vi "Run Tests.vi"(7 "Run Tests In Parallel? (T)":bool=TRUE, 8 "error in (no error)":errorcluster, 10 "Report Output path":path, 11 "Project, Library, or Test Class Path":path) -> (0 "error out":errorcluster, 1 "All Passed?":bool, 2 "Output":string)   [LabVIEW 2020, in "Execution API.lvclass"]
doc: "Run all tests from the selected path programmatically. The path may point to a .lvclass, .lvlib, or .lvproj file. Results are generated at the provided Report Output Path. If the file extenssion is .txt, a plain text file is generated, and if it is .xml, an JUnit compatible .xml report is generated."
uses:
  Execution API.lvclass
  Core/Result/Status.ctl
  Core/Result/Type.ctl
  Core/Result/Result.lvlib
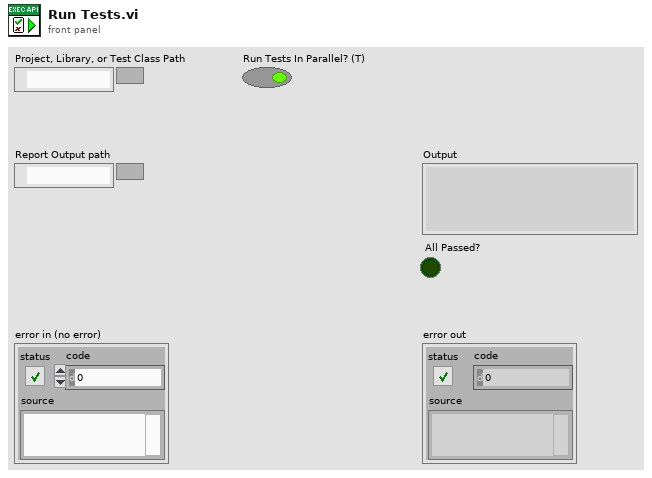
[diagram p1: front panel]
types:
  T1 = typedef "Result.lvlib/Status.ctl" = enum16{"", "Passed", "Failed", "Error", "Skipped", "Setup Error", "Broken", "Teardown Error"}
  T2 = typedef "Result.lvlib/Type.ctl" = enum16{"Test Case", "Test Suite", "Test Run", "Pass", "Fail", "Skip", "Pass if", "Fail if", "Pass if Error", "Fail if Error", "Pass if Equal", "Fail if Equal"}
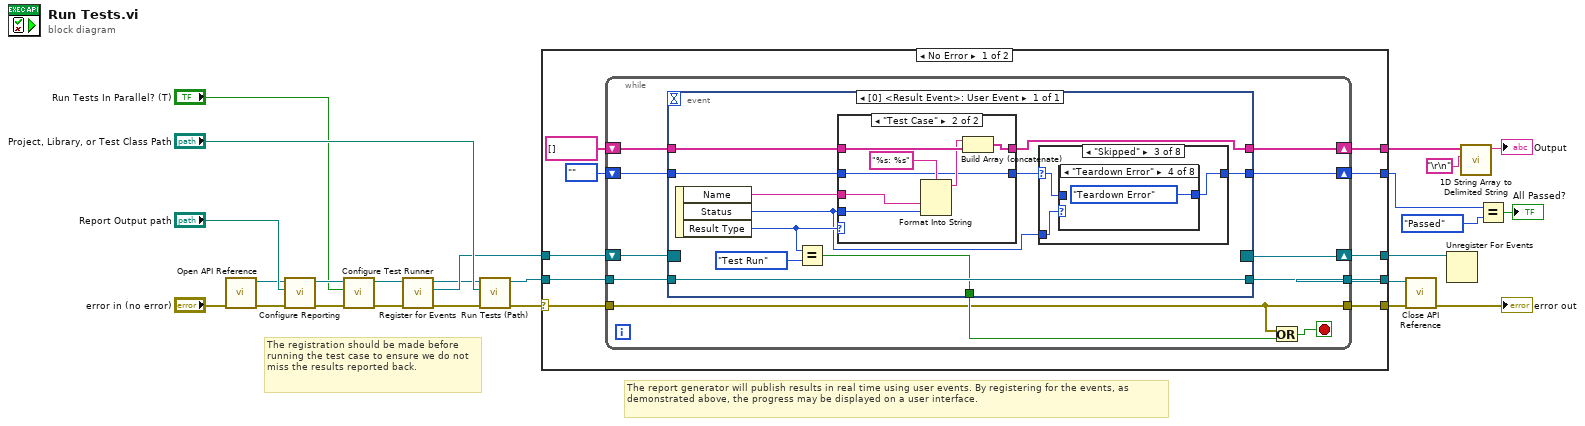
[diagram p0: block diagram]
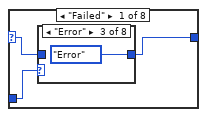
[diagram p3: hidden frame]
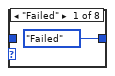
[diagram p4: hidden frame]
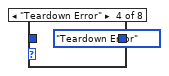
[diagram p6: hidden frame]
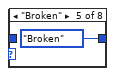
[diagram p7: hidden frame]
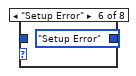
[diagram p8: hidden frame]
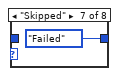
[diagram p9: hidden frame]
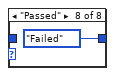
[diagram p10: hidden frame]
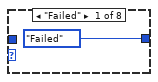
[diagram p12: hidden frame]
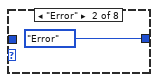
[diagram p13: hidden frame]
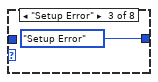
[diagram p14: hidden frame]
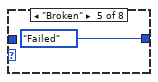
[diagram p15: hidden frame]
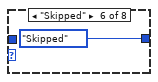
[diagram p16: hidden frame]
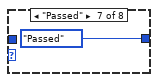
[diagram p17: hidden frame]
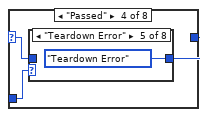
[diagram p19: hidden frame]
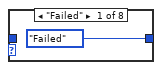
[diagram p20: hidden frame]
diagram:
  # "The registration should be made before running the test case to ensure we do not miss the results reported back."
  # "The report generator will publish results in real time using user events. By registering for the events, as demonstrated above, the progress may be displayed on a user interface."
  n1 = call "Open API Reference.vi"("error in (no error)"="error in (no error)") -> ("error out"=w13:errorcluster, "Execution API Out"=w17:refnum<class "Execution API.lvclass">)  [unwired: 9 in]
  n2 = call "Configure Reporting.vi"("error in (no error)"=w13, "Path"="Report Output path", "Execution API In"=w17) -> ("error out"=w15:errorcluster, "Execution API Out"=w14:refnum<class "Execution API.lvclass">)  [unwired: 7 in]
  n3 = call "Configure Test Runner.vi"("error in (no error)"=w15, "Run Tests In Parallel?"="Run Tests In Parallel? (T)", "Execution API In"=w14) -> ("error out"=w16:errorcluster, "Execution API Out"=w18:refnum<class "Execution API.lvclass">)  [unwired: 7 in]
  n4 = call "Register for Events.vi"("error in (no error)"=w16, "Execution API In"=w18) -> ("error out"=w10:errorcluster, "Event Registration"=w12:refnum<event-registration>, "Execution API Out"=w11:refnum<class "Execution API.lvclass">)  [unwired: 7 in]
  n5 = call "Run Tests (Path).vi"("error in (no error)"=w10, "Project or Class Path"="Project, Library, or Test Class Path", "Execution API In"=w11) -> ("error out"=w6:errorcluster, "Execution API Out"=w5:refnum<class "Execution API.lvclass">)  [unwired: 7 in]
  n6 = case shown="No Error" w6 {
    selector: w6 -> [w34 w115]
    tunnel: w12 -> [w35 w113]
    tunnel: w5 -> [w33 w114]
    tunnel: [w31 w115] -> w7
    tunnel: [w30 w114] -> w8
    tunnel: [w29 w113] -> w20
    tunnel: [w28 string[] []] -> w23
    tunnel: [w26 Status."Error" ("Status")] -> w3
    frame No Error {
      n7 = while {
        tunnel: w34 -> [w38]
        tunnel: w33 -> [w44]
        tunnel: [w42] -> w30
        tunnel: [w38] -> w31
        shift-right: [w39] -> w28
        shift-left: string[] [] -> [w46]
        shift-right: [w43] -> w29
        shift-left: w35 -> [w45]
        shift-right: [w36] -> w26
        shift-left: Status."" ("Status") -> [w37]
        stop <- w41 stop-if-true
        n8 = event shown="[0] <Result Event>: User Event" {
          selector: w45 -> [_]
          dyn-events: [_] -> w43
          timeout: _ -> [_]
          tunnel: w46 -> [w53]
          tunnel: w44 -> [w57]
          tunnel: [w57] -> w42
          tunnel: [w55] -> w40
          tunnel: [w52] -> w39
          tunnel: w37 -> [w50]
          tunnel: [w48] -> w36
          event User Event {
            n9 = event-data() -> ("Name"=w54:string, "Status"=w47:T1, "Result Type"=w51:T2)  [unwired: 1 in]
            n10 = Equal?(x=w51, y=Type."Test Run") -> (x = y?=w55:bool)
            n11 = case shown="\"Test Case\"" w51 {
              tunnel: w54 -> [_ w65]
              tunnel: w47 -> [_ w64]
              tunnel: w53 -> [w59 w63]
              tunnel: [w59 w61] -> w52
              tunnel: w50 -> [w58 w60]
              tunnel: [w58 w60] -> w49
              frame Default {
              }
              frame "Test Case" {
                n12 = Format Into String(format string="%s: %s", w65, w64) -> (resulting string=w62:string)  [unwired: 2 in, 1 out]
                n13 = Build Array (concatenate)(w62, w63) -> (w61:string[])
              }
            }
            n14 = case shown="\"Skipped\"" w49 {
              selector: w49 -> [w67 _ w79 w90 _ _ _ w108]
              tunnel: w47 -> [w69 w78 w81 w92 _ _ w103 _]
              tunnel: [w68 w78 w80 w91 Status."Error" ("Merged Status") Status."Setup Error" ("Merged Status") w104 w107] -> w48
              frame "Failed" {
                n15 = case shown="\"Error\"" w69 {
                  tunnel: [Status."Failed" ("Merged Status") w71 Status."Error" ("Merged Status") Status."Teardown Error" ("Merged Status") Status."Broken" ("Merged Status") Status."Setup Error" ("Merged Status") Status."Failed" ("Merged Status") Status."Failed" ("Merged Status")] -> w68
                  tunnel: w67 -> [_ w71 _ _ _ _ _ _]
                  frame "Failed" {
                  }
                  frame "" {
                  }
                  frame "Error" {
                  }
                  frame "Teardown Error" {
                  }
                  frame "Broken" {
                  }
                  frame "Setup Error" {
                  }
                  frame "Skipped" {
                  }
                  frame "Passed" {
                  }
                }
              }
              frame "" {
              }
              frame "Skipped" {
                n16 = case shown="\"Teardown Error\"" w81 {
                  tunnel: [Status."Failed" ("Merged Status") Status."Error" ("Merged Status") Status."Setup Error" ("Merged Status") Status."Teardown Error" ("Merged Status") Status."Failed" ("Merged Status") Status."Skipped" ("Merged Status") Status."Passed" ("Merged Status") w89] -> w80
                  tunnel: w79 -> [_ _ _ _ _ _ _ w89]
                  frame "Failed" {
                  }
                  frame "Error" {
                  }
                  frame "Setup Error" {
                  }
                  frame "Teardown Error" {
                  }
                  frame "Broken" {
                  }
                  frame "Skipped" {
                  }
                  frame "Passed" {
                  }
                  frame "" {
                  }
                }
              }
              frame "Passed" {
                n17 = case shown="\"Teardown Error\"" w92 {
                  tunnel: [Status."Failed" ("Merged Status") Status."Error" ("Merged Status") Status."Setup Error" ("Merged Status") Status."Failed" ("Merged Status") Status."Teardown Error" ("Merged Status") Status."Passed" ("Merged Status") w99 Status."Passed" ("Merged Status")] -> w91
                  tunnel: w90 -> [_ _ _ _ _ _ w99 _]
                  frame "Failed" {
                  }
                  frame "Error" {
                  }
                  frame "Setup Error" {
                  }
                  frame "Broken" {
                  }
                  frame "Teardown Error" {
                  }
                  frame "Skipped" {
                  }
                  frame "" {
                  }
                  frame "Passed" {
                  }
                }
              }
              frame "Error" {
              }
              frame "Setup Error" {
              }
              frame "Teardown Error" {
                n18 = case shown="Default" w103 {
                  selector: w103 -> [_ w106]
                  tunnel: [Status."Teardown Error" ("Merged Status") w106] -> w104
                  frame Default {
                  }
                  frame "Error", "Setup Error", "Broken" {
                  }
                }
              }
              frame "Broken" {
                n19 = case shown="\"Setup Error\"" w108 {
                  tunnel: [Status."Setup Error" ("New") Status."Broken" ("New")] -> w107
                  frame "Setup Error" {
                  }
                  frame Default {
                  }
                }
              }
            }
          }
        }
        n20 = Or(x=w38, y=w40) -> (x .or. y?=w41:bool)
      }
    }
    frame Error {
    }
  }
  n21 = call "Close API Reference.vi"("error in (no error)"=w7, "Execution API In"=w8) -> ("error out"=→"error out":errorcluster)  [unwired: 9 in]
  n22 = Unregister For Events(event registration refnum=w20) -> ()  [unwired: 1 in, 1 out]
  n23 = call <vilib>:"1D String Array to Delimited String.vi"("delimiter"="\r\n", "string array"=w23) -> ("delimited string"=→"Output":string)  [unwired: 9 in]
  n24 = Equal?(x=w3, y=Status."Passed" ("Status")) -> (x = y?=→"All Passed?":bool)
